vi "GetRxVoltage.vi"(6 "Legacy (f)?":bool, 8 "error in (no error)":errorcluster, 10 "Settling Time (0)":u32) -> (0 "error out":errorcluster, 2 "Rx, dBV":dbl)   [LabVIEW 2011]
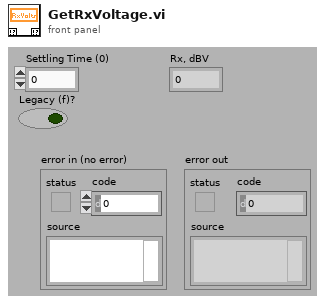
[diagram p1: front panel]
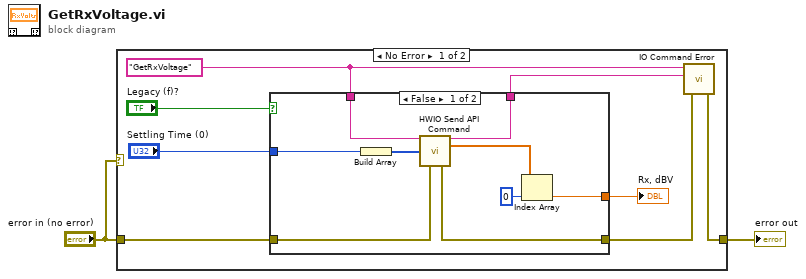
[diagram p0: block diagram]
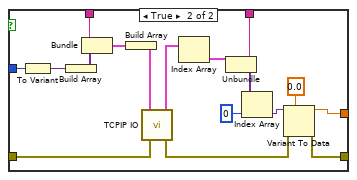
[diagram p2: hidden frame]
diagram:
  n1 = case shown="No Error" "error in (no error)" {
    tunnel: "error in (no error)" -> [w10 w37]
    tunnel: [w8 w37] -> w2
    frame No Error {
      w6 = "GetRxVoltage"
      n2 = case shown="False" "Legacy (f)?" {
        tunnel: w10 -> [w19 w35]
        tunnel: [w18 w33] -> w9
        tunnel: [w14 w32] -> w7
        tunnel: w6 -> [w13 w31]
        tunnel: [w15 w23] -> w5
        tunnel: "Settling Time (0)" -> [w12 w22]
        frame False {
          n3 = Build Array(w12) -> (w11:u32[])
          n4 = call "HWIO Send API Command.vi"("Action"=w13, "Integer"=w11, "error in (no error)"=w19) -> ("Action out"=w14:string, "Double out"=w17:dbl[], "error out"=w18:errorcluster)  [unwired: 5 in, 5 out]
          n5 = Index Array(array=w17, index=0) -> (element=w15:dbl)
        }
        frame True {
          n6 = To Variant(anything=w22) -> (Variant=w21:variant)
          n7 = Build Array(w21) -> (w20:variant[])
          n8 = Bundle(w31, w20) -> (w36:cluster{string, variant[]})  [unwired: 1 out]
          n9 = Build Array(w36) -> (w28:cluster{string, variant[]}[])
          n10 = call "TCPIP IO.vi"("error in (no error)"=w35, "Commands"=w28) -> ("error out"=w34:errorcluster, "Responses"=w30:cluster{string, variant[]}[])  [unwired: 1 in, 3 out]
          n11 = Index Array(array=w30) -> (element=w29:cluster{string, variant[]})  [unwired: 1 in]
          n12 = Unbundle(w29) -> (w32:string, w26:variant[])
          n13 = Index Array(array=w26, index=0) -> (element=w24:variant)
          n14 = Variant To Data(error in=w34, type=0.0, Variant=w24) -> (data=w23:dbl, error out=w33:errorcluster)
        }
      }
      "Rx, dBV" <- w5
      n15 = call "IO Command Error.vi"("error in (no error)"=w9, "Command Returned (\"\")"=w7, "Command Sent (\"\")"=w6) -> ("error out"=w8:errorcluster)  [unwired: 4 out]
    }
    frame Error {
    }
  }
  "error out" <- w2
